vi "Tests_misc.vi"   [LabVIEW 2024]
uses:
  <vilib>/Saukko/LV SDL3/Sources/SDL3/Video/Video.lvlib
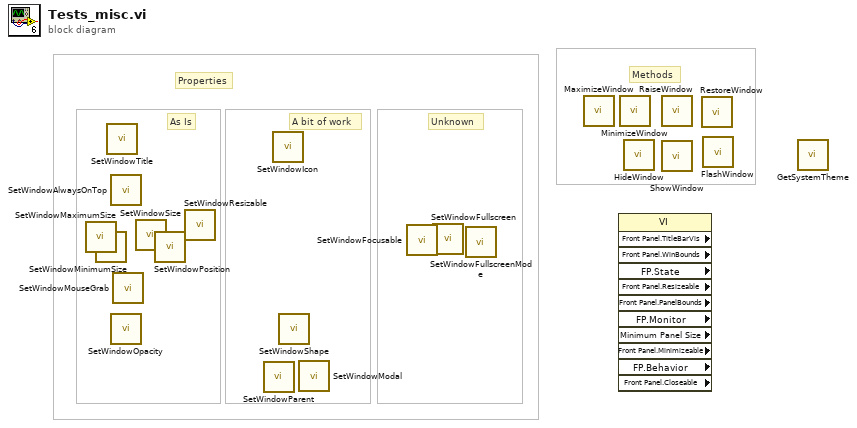
[diagram p0: block diagram]
diagram:
  # "Unknown"
  # "A bit of work"
  # "As Is"
  # "Properties"
  # "Methods"
  n1 = call <vilib>:"SetWindowMaximumSize.vi"() -> ()  [unwired: 11 in, 1 out]
  n2 = call <vilib>:"SetWindowMinimumSize.vi"() -> ()  [unwired: 11 in, 1 out]
  n3 = call <vilib>:"SetWindowTitle.vi"() -> ()  [unwired: 11 in, 1 out]
  n4 = call <vilib>:"SetWindowAlwaysOnTop.vi"() -> ()  [unwired: 11 in, 1 out]
  n5 = call <vilib>:"SetWindowOpacity.vi"() -> ()  [unwired: 11 in, 1 out]
  n6 = call <vilib>:"SetWindowMouseGrab.vi"() -> ()  [unwired: 11 in, 1 out]
  n7 = call <vilib>:"SetWindowSize.vi"() -> ()  [unwired: 11 in, 1 out]
  n8 = call <vilib>:"SetWindowPosition.vi"() -> ()  [unwired: 11 in, 1 out]
  n9 = call <vilib>:"SetWindowResizable.vi"() -> ()  [unwired: 11 in, 1 out]
  n10 = call <vilib>:"SetWindowParent.vi"() -> ()  [unwired: 11 in, 1 out]
  n11 = call <vilib>:"SetWindowIcon.vi"() -> ()  [unwired: 11 in, 1 out]
  n12 = call <vilib>:"SetWindowShape.vi"() -> ()  [unwired: 11 in, 1 out]
  n13 = call <vilib>:"SetWindowModal.vi"() -> ()  [unwired: 11 in, 1 out]
  n14 = call <vilib>:"SetWindowFocusable.vi"() -> ()  [unwired: 11 in, 1 out]
  n15 = call <vilib>:"SetWindowFullscreen.vi"() -> ()  [unwired: 11 in, 1 out]
  n16 = call <vilib>:"SetWindowFullscreenMode.vi"() -> ()  [unwired: 11 in, 1 out]
  n17 = call <vilib>:"MaximizeWindow.vi"() -> ()  [unwired: 11 in, 1 out]
  n18 = property class="VI" props=["Front Panel.TitleBarVis", "Front Panel.WinBounds", "FP.State", "Front Panel.Resizeable", "Front Panel.PanelBounds", "FP.Monitor", "Minimum Panel Size", "Front Panel.Minimizeable", "FP.Behavior", "Front Panel.Closeable"]() -> ()  [unwired: 2 in, 12 out]
  n19 = call <vilib>:"MinimizeWindow.vi"() -> ()  [unwired: 11 in, 1 out]
  n20 = call <vilib>:"HideWindow.vi"() -> ()  [unwired: 11 in, 1 out]
  n21 = call <vilib>:"RaiseWindow.vi"() -> ()  [unwired: 11 in, 1 out]
  n22 = call <vilib>:"ShowWindow.vi"() -> ()  [unwired: 11 in, 1 out]
  n23 = call <vilib>:"RestoreWindow.vi"() -> ()  [unwired: 11 in, 1 out]
  n24 = call <vilib>:"FlashWindow.vi"() -> ()  [unwired: 11 in, 1 out]
  n25 = call <vilib>:"GetSystemTheme.vi"() -> ()  [unwired: 10 in, 2 out]
